vi "LEDC SWIR 1931 Init.vi"(0 "LEDAD Port":refnum<visa-resource-name>="COM7", 1 "Wavelength":string, 5 "Light Meter Port":refnum<visa-resource-name>="COM4", 11 "error in (no error)":errorcluster) -> (3 "In Progress":bool, 4 "LEDAD Port out":refnum<visa-resource-name>, 6 "Light Meter Port out":refnum<visa-resource-name>, 14 "Done":bool, 15 "error out":errorcluster)   [LabVIEW 2010]
panel:
  # "nm"
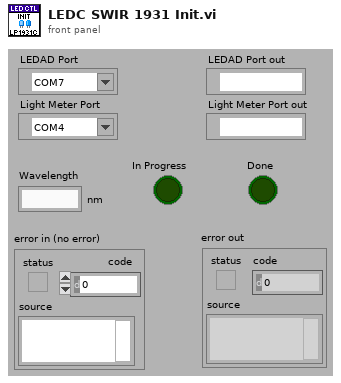
[diagram p1: front panel]
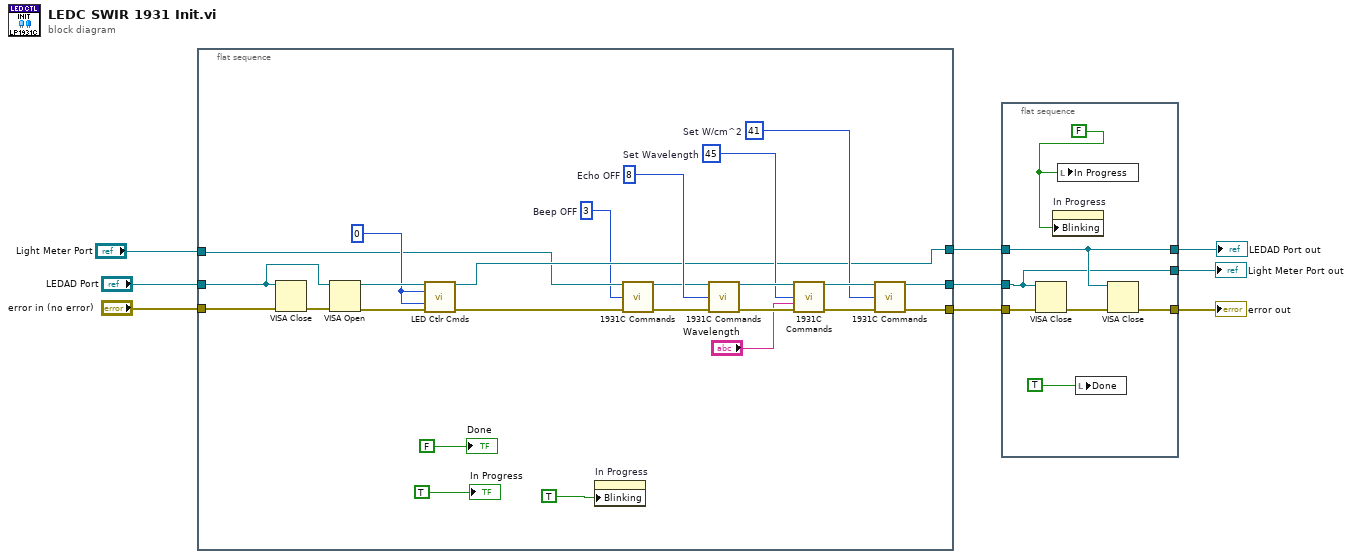
[diagram p0: block diagram]
diagram:
  n1 = flat-sequence {
    tunnel: "error in (no error)" -> [w34]
    tunnel: "LEDAD Port" -> [w32]
    tunnel: "Light Meter Port" -> [w14]
    tunnel: [w20] -> w2
    tunnel: [w19] -> w3
    tunnel: [w16] -> w1
    frame #0 {
      w10 = 3  # Beep OFF
      w22 = 41  # Set W/cm^2
      w28 = 45  # Set Wavelength
      w31 = 8  # Echo OFF
      w15 = 0
      n2 = VISA Close(VISA resource name=w32, error in (no error)=w34) -> (error out=w33:errorcluster)
      n3 = VISA Open(error in (no error)=w33, VISA resource name=w32) -> (VISA resource name=w18:refnum<visa-resource-name>, error out=w17:errorcluster)  [unwired: 3 in]
      n4 = call "LED Ctlr Cmds.vi"("VISA session"=w18, "Intensity"=w15, "Enable"=w15, "error in (no error)"=w17) -> ("VISA session out"=w16:refnum<visa-resource-name>, "error out"=w13:errorcluster)  [unwired: 7 in, 3 out]
      n5 = property on="In Progress" class="Bool (strict)"("Blinking"=TRUE) -> ()  [unwired: 2 in, 2 out]
      n6 = call "1931C Commands.vi"("Instrument Resource Name"=w14, "Command"=w10, "error in (no error)"=w13) -> ("VISA resource name out"=w12:refnum<visa-resource-name>, "error out"=w11:errorcluster)  [unwired: 8 in, 3 out]
      n7 = call "1931C Commands.vi"("Instrument Resource Name"=w12, "Command"=w31, "error in (no error)"=w11) -> ("VISA resource name out"=w29:refnum<visa-resource-name>, "error out"=w30:errorcluster)  [unwired: 8 in, 3 out]
      n8 = call "1931C Commands.vi"("Instrument Resource Name"=w29, "Command"=w28, "Wavelength"="Wavelength", "error in (no error)"=w30) -> ("VISA resource name out"=w23:refnum<visa-resource-name>, "error out"=w24:errorcluster)  [unwired: 7 in, 3 out]
      n9 = call "1931C Commands.vi"("Instrument Resource Name"=w23, "Command"=w22, "error in (no error)"=w24) -> ("VISA resource name out"=w20:refnum<visa-resource-name>, "error out"=w19:errorcluster)  [unwired: 8 in, 3 out]
      "Done" <- FALSE
      "In Progress" <- TRUE
    }
  }
  n10 = flat-sequence {
    tunnel: w2 -> [w37]
    tunnel: w3 -> [w39]
    tunnel: [w38] -> w4
    tunnel: w1 -> [w38]
    tunnel: [w37] -> w5
    tunnel: [w35] -> w6
    frame #0 {
      w41 = FALSE
      n11 = VISA Close(VISA resource name=w37, error in (no error)=w39) -> (error out=w36:errorcluster)
      n12 = property on="In Progress" class="Bool (strict)"("Blinking"=w41) -> ()  [unwired: 2 in, 2 out]
      n13 = local write "In Progress"(w41) -> ()
      n14 = local write "Done"(TRUE) -> ()
      n15 = VISA Close(VISA resource name=w38, error in (no error)=w36) -> (error out=w35:errorcluster)
    }
  }
  "LEDAD Port out" <- w4
  "Light Meter Port out" <- w5
  "error out" <- w6
